vi "Channel Scale Map.vi"(7 "Channels":string[](array[string]), 10 "Chart Scales":T1, 11 "Chart in":refnum<vi>) -> (2 "Channel Scale Map":map{string, string}(c390), 3 "Chart":refnum<vi>)   [LabVIEW 2020, in "VolatusGUIControls.lvlib" / "SimpleGraphEditorPanel.lvclass"]
uses:
  SimpleGraphEditorPanel.lvclass
  SimpleGraphEditorPanel.lvclass/SimpleGraphEditorPanel.ctl
  VolatusGUIEditorCore/Chart Scale Props.ctl
  VolatusGUIEditorCore/VolatusGUIEditorCore.lvlib
  VolatusGUIEditorCore/Chart Scales.ctl
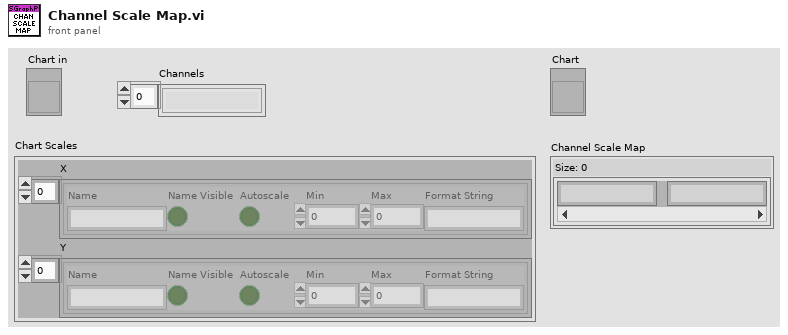
[diagram p1: front panel]
types:
  T1 = typedef "VolatusGUIEditorCore.lvlib/Chart Scales.ctl" = cluster{"X":T2[], "Y":T2[]}
  T2 = typedef "VolatusGUIEditorCore.lvlib/Chart Scale Props.ctl" = cluster{"Name":string, "Name Visible":bool, "Autoscale":bool, "Min":dbl, "Max":dbl, "Format String":string}
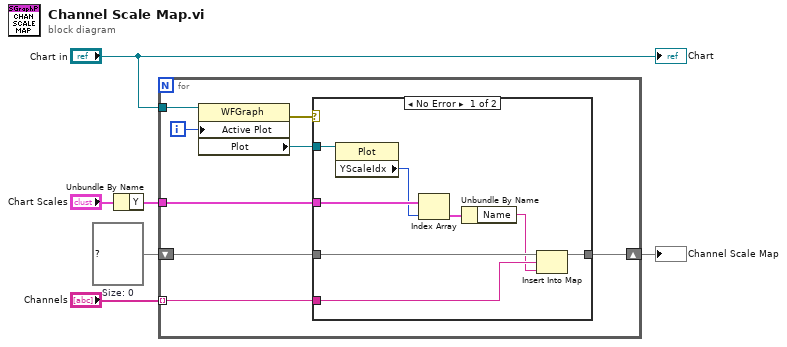
[diagram p0: block diagram]
diagram:
  w5 = map{string, string} {}  # Size: 0
  n1 = Unbundle By Name("Chart Scales") -> ("Y"=w3:T2[])
  n2 = for {
    tunnel: "Channels" -> [w8] mode=indexing
    shift-right: [w7] -> w2
    shift-left: w5 -> [w9]
    tunnel: w3 -> [w10]
    tunnel: "Chart in" -> [w14]
    i -> [w13]
    n3 = property class="WFGraph"(reference=w14, "Active Plot"=w13) -> (error out=w11:errorcluster, "Plot"=w12:refnum<vi>)  [unwired: 1 in, 1 out]
    n4 = case shown="No Error" w11 {
      tunnel: w12 -> [w22 _]
      tunnel: w10 -> [w21 _]
      tunnel: w9 -> [w18 w23]
      tunnel: w8 -> [w17 _]
      tunnel: [w15 w23] -> w7
      frame No Error {
        n5 = property class="Plot"(reference=w22) -> ("YScaleIdx"=w20:u32)  [unwired: 1 in, 2 out]
        n6 = Index Array(array=w21, index=w20) -> (element=w19:T2)
        n7 = Unbundle By Name(w19) -> ("Name"=w16:string)
        n8 = Insert Into Map(map in=w18, key=w17, value=w16) -> (map out=w15:map{string, string})  [unwired: 2 out]
      }
      frame Error {
      }
    }
  }
  "Channel Scale Map" <- w2
  "Chart" <- "Chart in"
